vi "52 Properties.vi"() -> ()   [LabVIEW 2024]
uses:
  <userlib>/1. Examples/_Subs/OpenDiagram/Open_XControl.xctl
panel:
  in  "OpenDiag":refnum<vi>(xcontrol)
  in  "Mess":bool
  out "Waveform Graph":dbl[](graph)
  in  "Stop Button":bool
  out "Choice":string
  in  "Menu of Choices":u16(ring) items=["Old", "Medium", "Young", "Baby"]
  # "02 Properties\nThis code uses properties to programmatically change things on the front panel\n\nInstructions:\n1. Hit the Run arrow and Select a choice.  Notice in the diagram how the choices populated"
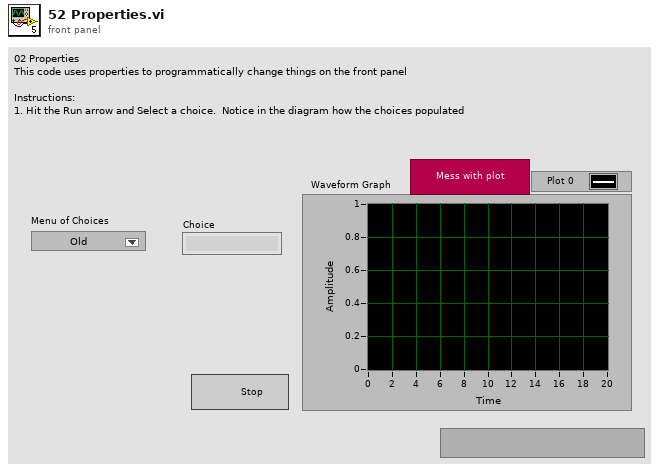
[diagram p1: front panel]
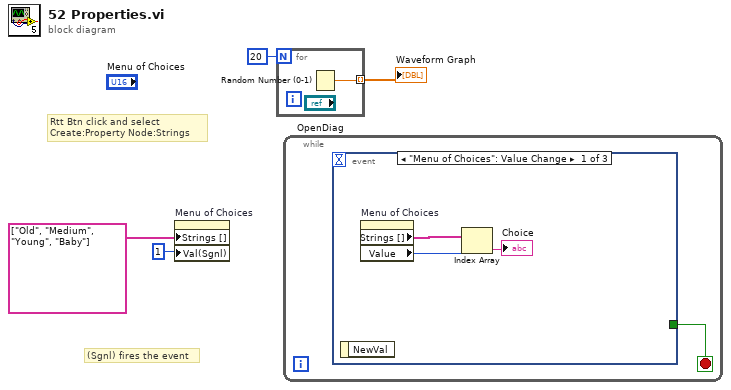
[diagram p0: block diagram]
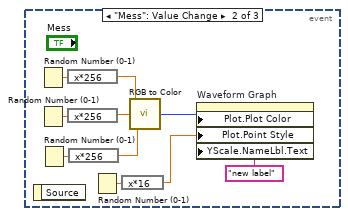
[diagram p2: hidden frame]
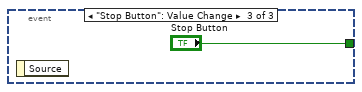
[diagram p3: hidden frame]
diagram:
  # "Rtt Btn click and select\nCreate:Property Node:Strings"
  # "(Sgnl) fires the event"
  n1 = property on="Menu of Choices" class="Ring (strict)"("Strings []"=string[] ["Old", "Medium", "Young", "Baby"], "Val(Sgnl)"=u16 1 ("Value (Signaling)")) -> ()  [unwired: 2 in, 2 out]
  n2 = for {
    N: 20 -> [_]
    tunnel: [w5] -> w1 mode=indexing
    n3 = Random Number (0-1)() -> (number: 0 to 1=w5:dbl)
  }
  "Waveform Graph" <- w1
  n4 = while {
    stop <- w6 stop-if-true
    n5 = event shown="[0] \"Menu of Choices\": Value Change" {
      selector: _ -> [_ _ _]
      dyn-events: _ -> [_ _ _]
      timeout: _ -> [_ _ _]
      tunnel: [_ _ "Stop Button"] -> w6
      event "Menu of Choices": Value Change {
        n6 = event-data() -> ()  [unwired: 1 in, 1 out]
        n7 = property on="Menu of Choices" class="Ring (strict)"() -> ("Strings []"=w8:string[], "Value"=w9:u16)  [unwired: 2 in, 2 out]
        n8 = Index Array(array=w8, index=w9) -> (element=→"Choice":string)
      }
      event "Mess": Value Change {
        n9 = event-data() -> ()  [unwired: 1 in, 1 out]
        n10 = Random Number (0-1)() -> (number: 0 to 1=w17:dbl)
        n11 = Random Number (0-1)() -> (number: 0 to 1=w16:dbl)
        n12 = Random Number (0-1)() -> (number: 0 to 1=w15:dbl)
        n13 = expression code="x*256"(w17) -> (w18:dbl)
        n14 = expression code="x*256"(w16) -> (w13:dbl)
        n15 = expression code="x*256"(w15) -> (w14:dbl)
        n16 = Random Number (0-1)() -> (number: 0 to 1=w12:dbl)
        n17 = expression code="x*16"(w12) -> (w11:dbl)
        n18 = call <vilib>:"RGB to Color.vi"("B"=w14, "G"=w13, "R"=w18) -> ("Color"=w19:u32)
        n19 = property on="Waveform Graph" class="WFGraph (strict)"("Plot.Plot Color"=w19, "Plot.Point Style"=w11, "YScale.NameLbl.Text"="new label" ("Y Scale.Name Label.Text")) -> ()  [unwired: 2 in, 2 out]
      }
      event "Stop Button": Value Change {
        n20 = event-data() -> ()  [unwired: 1 in, 1 out]
      }
    }
  }
